vi "GetFPGAdispValues_v2.vi"(8 "error in (no error)":errorcluster, 11 "FPGA VI Reference In":T1) -> (0 "error out":errorcluster, 2 "State variables":dbl[](array[numeric]), 3 "FPGA VI Reference Out":T1)   [LabVIEW 2017]
doc: "Get values for display from FPGA."
uses:
  <vilib>/rvi/interface/nirviReadWriteControl/nirviReadWriteControl.xnode
  TypeDefs/FPGA VI Reference.ctl
  FPGA Bitfiles/flexlab_FPGATarget_Tbeamrawv2MainVI_U8ISWGKWIPM.lvbitx
  NiFpgaLv.dll
  <vilib>/Utility/error.llb/Error Cluster From Error Code.vi
  <vilib>/rvi/errors/niLvFpgaAdjustHostInterfaceError.vi
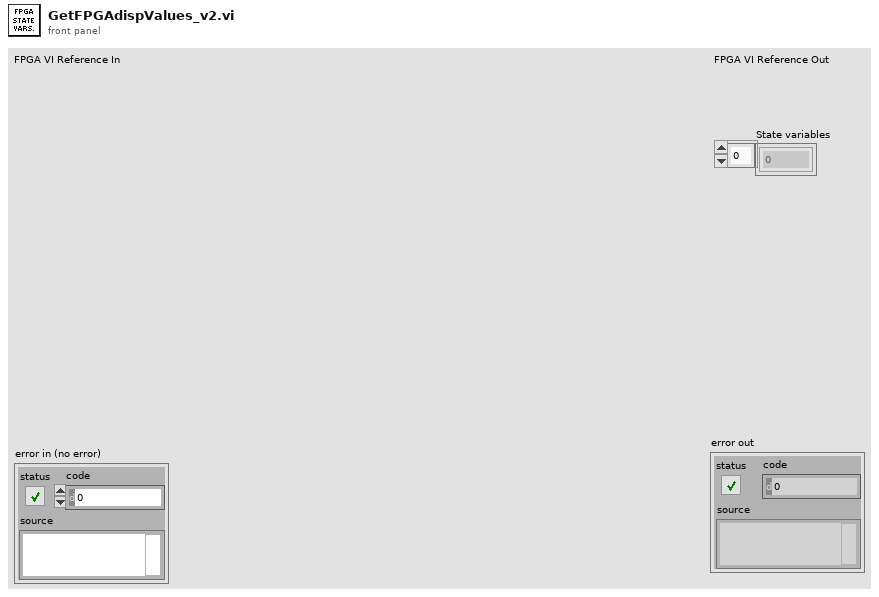
[diagram p1: front panel]
types:
  T1 = typedef "FPGA VI Reference.ctl" = refnum<k20>
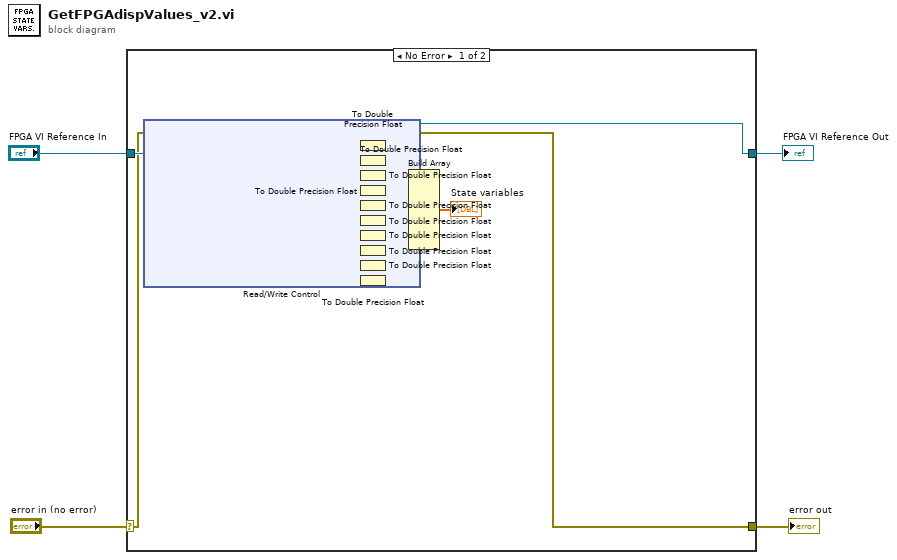
[diagram p0: block diagram]
diagram:
  n1 = case shown="No Error" "error in (no error)" {
    selector: "error in (no error)" -> [w12 w31]
    tunnel: [w11 w31] -> w3
    tunnel: [w13 w30] -> w1
    tunnel: "FPGA VI Reference In" -> [w29 w30]
    frame No Error {
      n2 = xnode "Read/Write Control"("FPGA VI Reference In"=w29, "error in"=w12) -> ("FPGA VI Reference Out"=w13:T1, "error out"=w11:errorcluster, "Bend reference [V]"=w8:fxp<+/-,25,4>, "Twist reference [V]"=w7:fxp<+/-,25,4>, "Bend [V]"=w21:fxp<+/-,25,4>, "Twist [V]"=w20:fxp<+/-,25,4>, "Hall2 [V]"=w19:fxp<+,25,3>, "Hall3 [V]"=w18:fxp<+,25,3>, "U_bend [V]"=w17:fxp<+/-,26,4>, "U_twist [V]"=w16:fxp<+/-,26,4>, "AO Coil2 [V]"=w15:fxp<+,25,3>, "AO Coil3 [V]"=w14:fxp<+,25,3>)
      n3 = To Double Precision Float(number=w8) -> (double precision float=w5:dbl)
      n4 = To Double Precision Float(number=w7) -> (double precision float=w6:dbl)
      n5 = To Double Precision Float(number=w21) -> (double precision float=w9:dbl)
      n6 = To Double Precision Float(number=w20) -> (double precision float=w22:dbl)
      n7 = To Double Precision Float(number=w19) -> (double precision float=w23:dbl)
      n8 = To Double Precision Float(number=w18) -> (double precision float=w28:dbl)
      n9 = To Double Precision Float(number=w17) -> (double precision float=w27:dbl)
      n10 = To Double Precision Float(number=w16) -> (double precision float=w26:dbl)
      n11 = To Double Precision Float(number=w15) -> (double precision float=w24:dbl)
      n12 = To Double Precision Float(number=w14) -> (double precision float=w25:dbl)
      n13 = Build Array(w5, w6, w9, w22, w23, w28, w27, w26, w24, w25) -> (→"State variables":dbl[])
    }
    frame Error {
    }
  }
  "error out" <- w3
  "FPGA VI Reference Out" <- w1
